vi "Create Server Library from Template.vi"(8 "error in (no error)":errorcluster, 9 "Generated Server Name":string="Generated Server", 10 "Target Project Path":path, 11 "Application ref in":refnum<vi>) -> (0 "error out":errorcluster, 3 "Server library out":refnum<vi>)   [LabVIEW 2020, in "gRPC Template Creation Utility.lvlib"]
uses:
  gRPC Template Creation Utility.lvlib
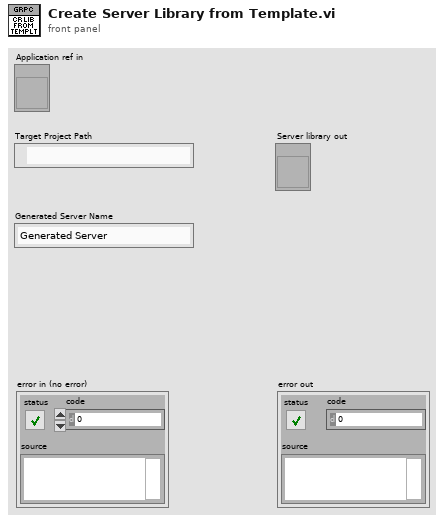
[diagram p1: front panel]
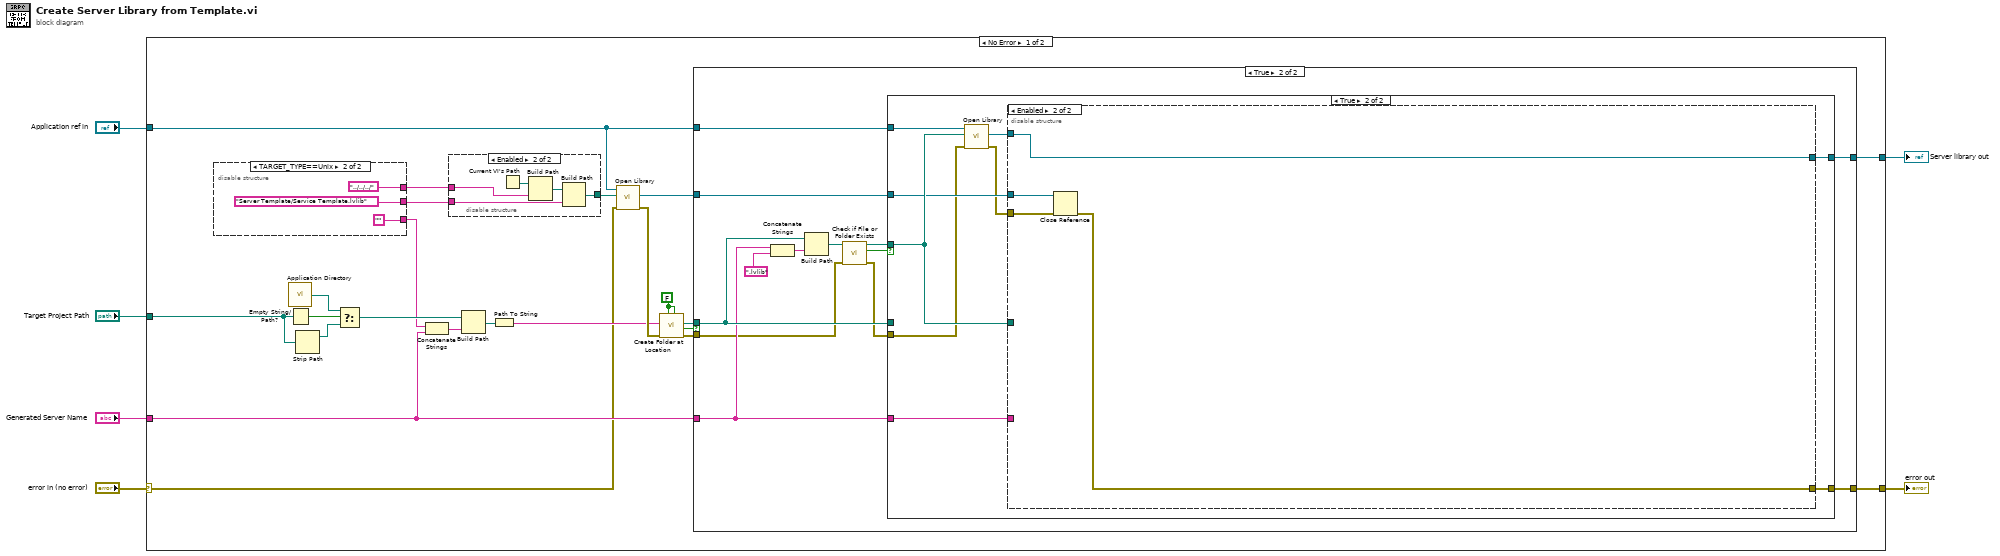
[diagram p0: block diagram]
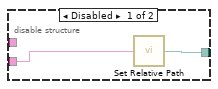
[diagram p2: hidden frame]
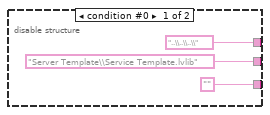
[diagram p3: hidden frame]
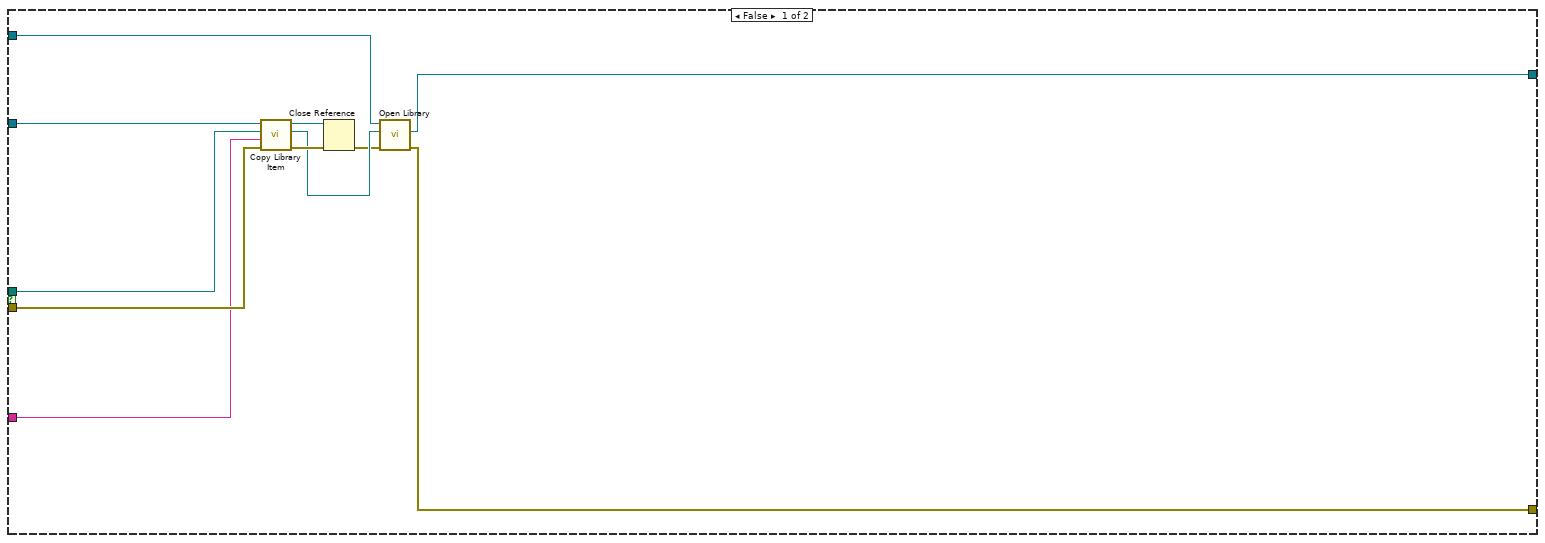
[diagram p4: hidden frame]
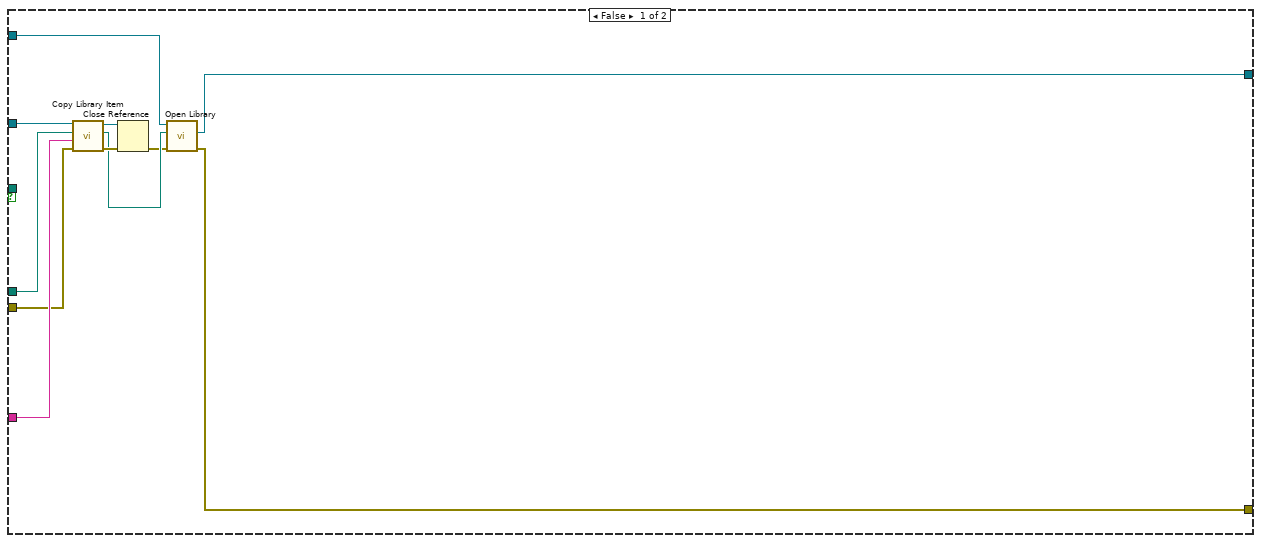
[diagram p5: hidden frame]
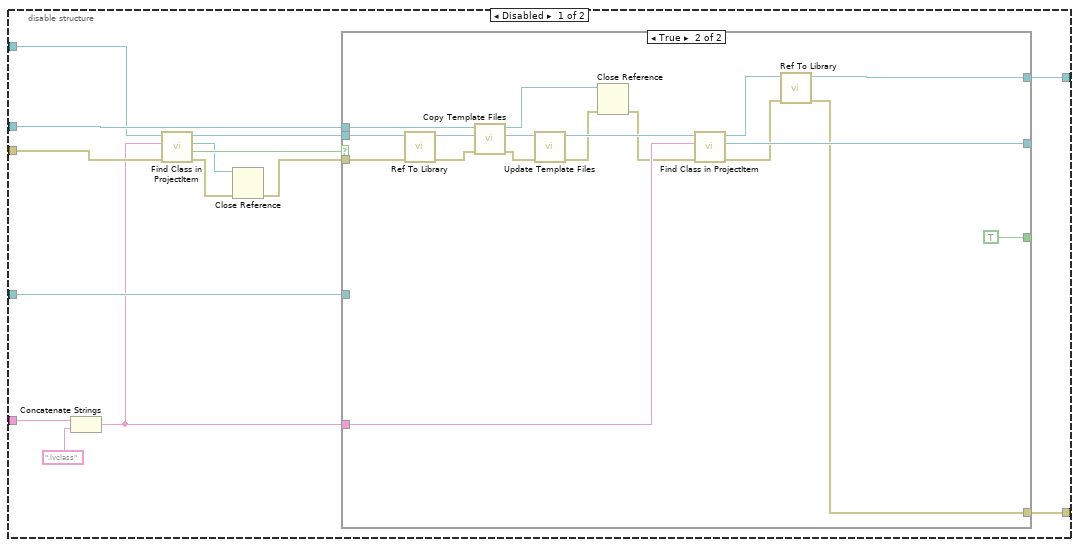
[diagram p6: hidden frame]
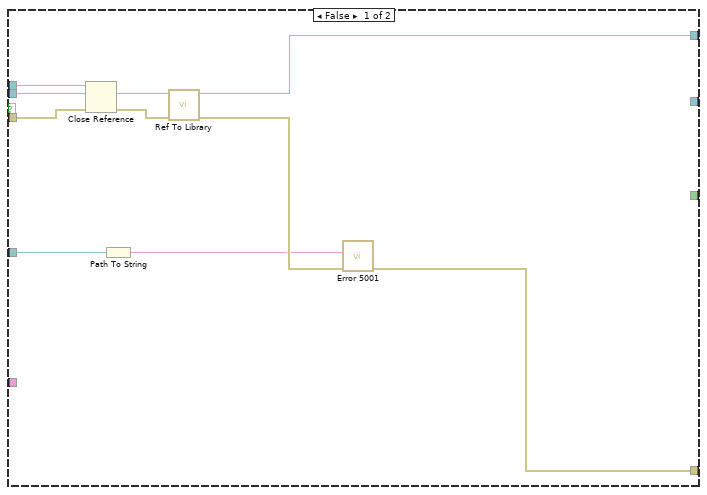
[diagram p7: hidden frame]
diagram:
  n1 = case shown="No Error" "error in (no error)" {
    selector: "error in (no error)" -> [w11 w132]
    tunnel: [w29 w132] -> w6
    tunnel: [w28 _] -> w5
    tunnel: "Target Project Path" -> [w14 _]
    tunnel: "Generated Server Name" -> [w13 _]
    tunnel: "Application ref in" -> [w12 _]
    frame No Error {
      w22 = FALSE ("Use Relative")
      n2 = disable-structure shown="TARGET_TYPE==Unix" {
        disable-tunnel: ["Server Template\\Service Template.lvlib" ("Application Relative Path") "Server Template/Service Template.lvlib" ("Application Relative Path")] -> w9
        disable-tunnel: ["" ("Path") "" ("Path")] -> w8
        disable-tunnel: ["..\\..\\..\\" ("name or relative path") "../../../" ("name or relative path")] -> w7
        frame condition #0 {
        }
        frame condition #1 (active) {
        }
      }
      n3 = call <vilib>:"Application Directory.vi"() -> ("Application Directory"=w15:path)
      n4 = Empty String/Path?(string/path=w14) -> (empty?=w18:bool)
      n5 = Strip Path(path=w14) -> (stripped path=w17:path)  [unwired: 1 out]
      n6 = Select(t=w15, s=w18, f=w17) -> (s? t:f=w16:path)
      n7 = Concatenate Strings(w8, w13) -> (w21:string)
      n8 = disable-structure shown="Enabled" {
        disable-tunnel: [w31 w35] -> w25
        disable-tunnel: w9 -> [w30 w33]
        disable-tunnel: w7 -> [_ w32]
        frame Disabled {
          n9 = call "Set Relative Path.vi"("Application Relative Path"=w30) -> ("Full Path"=w31:path)
        }
        frame Enabled {
          n10 = Current VI's Path() -> (path=w36:path)
          n11 = Build Path(base path=w36, name or relative path=w32) -> (appended path=w34:path)
          n12 = Build Path(base path=w34, name or relative path=w33) -> (appended path=w35:path)
        }
      }
      n13 = Build Path(base path=w16, name or relative path=w21) -> (appended path=w20:path)
      n14 = Path To String(path=w20) -> (string=w19:string)
      n15 = call "Open Library.vi"("error in (no error)"=w11, "Full Path"=w25, "Application in"=w12) -> ("error out"=w26:errorcluster, "Library out"=w23:refnum<vi>)  [unwired: 6 in, 1 out]
      n16 = call "Create Folder at Location.vi"("Override existing (F)"=w22, "Use Relative (F)"=w22, "Error In"=w26, "Path"=w19) -> ("Error Out"=w27:errorcluster, "Already Exists ?"=w10:bool, "Full path out"=w24:path)  [unwired: 5 in]
      n17 = case shown="True" w10 {
        tunnel: [w45 w57] -> w29
        tunnel: [w53 w62] -> w28
        tunnel: w27 -> [w50 w55]
        tunnel: w24 -> [w49 w59]
        tunnel: w23 -> [w48 w60]
        tunnel: w13 -> [w44 w58]
        tunnel: w12 -> [w43 w61]
        frame False {
          n18 = call "Copy Library Item.vi"("error in (no error)"=w50, "Copy Name"=w44, "Copy location"=w49, "Library in"=w48) -> ("error out"=w52:errorcluster, "New Lib Path"=w47:path, "Library out"=w51:refnum<vi>)  [unwired: 5 in]
          n19 = Close Reference(reference=w51, error in (no error)=w52) -> (error out=w46:errorcluster)
          n20 = call "Open Library.vi"("error in (no error)"=w46, "Full Path"=w47, "Application in"=w43) -> ("error out"=w45:errorcluster, "Library out"=w53:refnum<vi>)  [unwired: 6 in, 1 out]
        }
        frame True {
          n21 = Concatenate Strings(w58, ".lvlib" ("string")) -> (w65:string)
          n22 = Build Path(base path=w59, name or relative path=w65) -> (appended path=w64:path)
          n23 = call <vilib>:"Check if File or Folder Exists.vi"("error in (no error)"=w55, "path"=w64) -> ("error out"=w54:errorcluster, "file or folder exists?"=w63:bool, "dup path"=w56:path)  [unwired: 7 in]
          n24 = case shown="True" w63 {
            tunnel: [w72 w84] -> w62
            tunnel: w61 -> [w71 w86]
            tunnel: w60 -> [w70 w81]
            tunnel: w59 -> [w69 _]
            tunnel: w58 -> [w68 w85]
            tunnel: w54 -> [w67 w80]
            tunnel: [w73 w83] -> w57
            tunnel: w56 -> [_ w82]
            frame False {
              n25 = call "Copy Library Item.vi"("error in (no error)"=w67, "Copy Name"=w68, "Copy location"=w69, "Library in"=w70) -> ("error out"=w77:errorcluster, "New Lib Path"=w75:path, "Library out"=w76:refnum<vi>)  [unwired: 5 in]
              n26 = Close Reference(reference=w76, error in (no error)=w77) -> (error out=w74:errorcluster)
              n27 = call "Open Library.vi"("error in (no error)"=w74, "Full Path"=w75, "Application in"=w71) -> ("error out"=w73:errorcluster, "Library out"=w72:refnum<vi>)  [unwired: 6 in, 1 out]
            }
            frame True {
              n28 = call "Open Library.vi"("error in (no error)"=w80, "Full Path"=w82, "Application in"=w86) -> ("error out"=w78:errorcluster, "Library out"=w79:refnum<vi>)  [unwired: 6 in, 1 out]
              n29 = disable-structure shown="Enabled" {
                disable-tunnel: w85 -> [w100 _]
                disable-tunnel: [w99 w131] -> w84
                disable-tunnel: [w98 w128] -> w83
                disable-tunnel: w82 -> [w97 _]
                disable-tunnel: w81 -> [w96 w130]
                disable-tunnel: w79 -> [w95 w131]
                disable-tunnel: w78 -> [w93 w129]
                frame Disabled {
                  n30 = Concatenate Strings(w100, ".lvclass" ("Class Name")) -> (w87:string)
                  n31 = call "Find Class in ProjectItem.vi"("error in (no error)"=w93, "Class Name"=w87, "ProjectItem in"=w95) -> ("error out"=w89:errorcluster, "Found?"=w91:bool, "LVClass out"=w90:refnum<vi>, "ProjectItem out"=w92:refnum<vi>)  [unwired: 5 in]
                  n32 = Close Reference(reference=w90, error in (no error)=w89) -> (error out=w88:errorcluster)
                  n33 = case shown="True" w91 {
                    tunnel: w92 -> [w109 w122]
                    tunnel: [w108 w127] -> w99
                    tunnel: w88 -> [w103 w124]
                    tunnel: [w106 w115] -> w98
                    tunnel: w97 -> [w105 _]
                    tunnel: [_ TRUE] -> _
                    tunnel: w96 -> [w104 w114]
                    tunnel: w87 -> [_ w121]
                    tunnel: [_ w120] -> _
                    frame False {
                      n34 = Close Reference(reference=w104, error in (no error)=w103) -> (error out=w102:errorcluster)
                      n35 = Path To String(path=w105) -> (string=w101:string)
                      n36 = call "Ref To Library.vi"("error in (no error)"=w102, "ProjectItem in"=w109) -> ("error out"=w107:errorcluster, "Library out"=w108:refnum<vi>)  [unwired: 8 in]
                      n37 = call "Error 5001.vi"("error in (no error)"=w107, "Server Class Path"=w101) -> ("error out"=w106:errorcluster)  [unwired: 9 in]
                    }
                    frame True {
                      n38 = call "Ref To Library.vi"("error in (no error)"=w124, "ProjectItem in"=w122) -> ("error out"=w123:errorcluster, "Library out"=w125:refnum<vi>)  [unwired: 8 in]
                      n39 = call "Copy Template Files.vi"("error in (no error)"=w123, "Server Library (Library Item) in"=w125, "Template Library (Library Item) in"=w114) -> ("error out"=w113:errorcluster, "Server Library (Library Item) out"=w112:refnum<vi>, "Template Library (Library Item) out"=w110:refnum<vi>)  [unwired: 6 in]
                      n40 = call "Update Template Files.vi"("error in (no error)"=w113, "Server Library (Library Item) in"=w112) -> ("error out"=w111:errorcluster, "Server Library (Library Item) out"=w119:refnum<vi>)  [unwired: 8 in]
                      n41 = Close Reference(reference=w110, error in (no error)=w111) -> (error out=w117:errorcluster)
                      n42 = call "Find Class in ProjectItem.vi"("error in (no error)"=w117, "Class Name"=w121, "ProjectItem in"=w119) -> ("error out"=w116:errorcluster, "LVClass out"=w120:refnum<vi>, "ProjectItem out"=w118:refnum<vi>)  [unwired: 5 in, 1 out]
                      n43 = call "Ref To Library.vi"("error in (no error)"=w116, "ProjectItem in"=w118) -> ("error out"=w115:errorcluster, "Library out"=w127:refnum<vi>)  [unwired: 8 in]
                    }
                  }
                }
                frame Enabled {
                  n44 = Close Reference(reference=w130, error in (no error)=w129) -> (error out=w128:errorcluster)
                }
              }
            }
          }
        }
      }
    }
    frame Error {
    }
  }
  "error out" <- w6
  "Server library out" <- w5
